vi "Reset_To_Default.vi"(8 "error in (no error)":errorcluster, 11 "MHL_Data In":T1) -> (0 "error out":errorcluster, 3 "MHL_Data Out":T1)   [LabVIEW 2019, in "MHL.lvlib"]
uses:
  MHL.lvlib
  typedef/MHL_Data.ctl
  Alarm_Panel/Channel_Temperature_Threshold.ctl
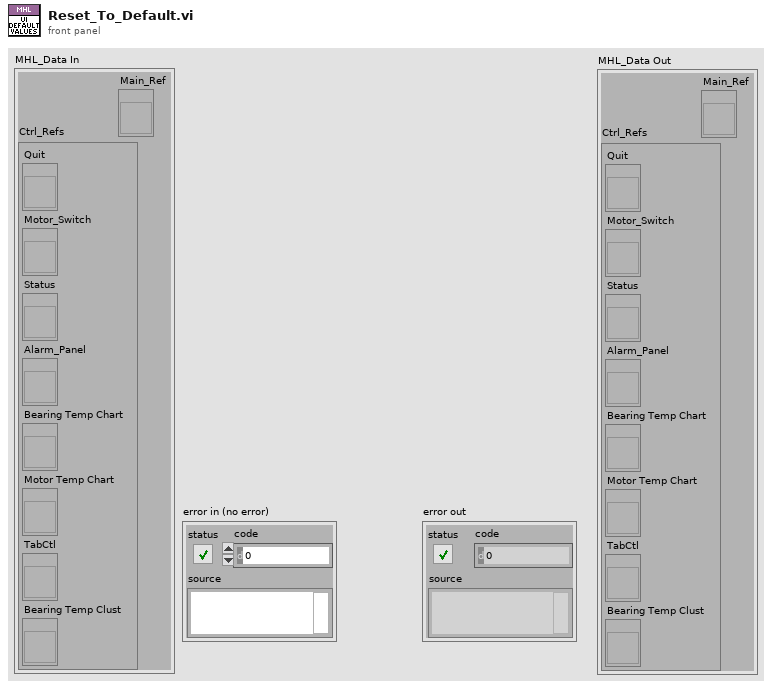
[diagram p1: front panel]
types:
  T1 = typedef "MHL.lvlib/MHL_Data.ctl" = cluster{"Ctrl_Refs":cluster{"Quit":refnum<vi>, "Motor_Switch":refnum<vi>, "Status":refnum<vi>, "Alarm_Panel":refnum<vi>, "Bearing Temp Chart":refnum<vi>, "Motor Temp Chart":refnum<vi>, "TabCtl":refnum<vi>, "Bearing Temp Clust":refnum<vi>}, "Main_Ref":refnum<vi>}
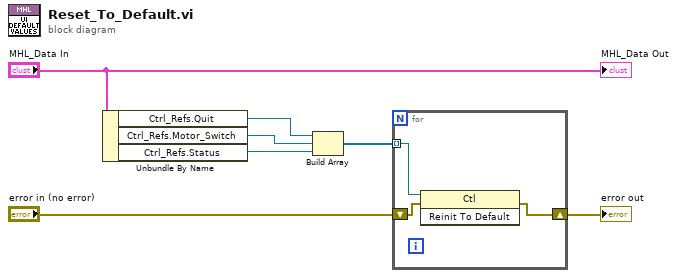
[diagram p0: block diagram]
diagram:
  n1 = Unbundle By Name("MHL_Data In") -> ("Ctrl_Refs.Quit"=w5:refnum<vi>, "Ctrl_Refs.Motor_Switch"=w6:refnum<vi>, "Ctrl_Refs.Status"=w7:refnum<vi>)
  n2 = Build Array(w5, w6, w7) -> (w4:refnum<vi>[])
  n3 = for {
    tunnel: w4 -> [w10] mode=indexing
    shift-right: [w8] -> w2
    shift-left: "error in (no error)" -> [w9]
    n4 = invoke class="Ctl" method="Reinit To Default"(reference=w10, error in=w9) -> (error out=w8:errorcluster)  [unwired: 1 in, 2 out]
  }
  "error out" <- w2
  "MHL_Data Out" <- "MHL_Data In"
